vi "Save Documentation to VIs.vi"(8 "error in":errorcluster, 10 "VI Information Array":T1[](array[typedef]), 11 "Engine in":refnum<class "Engine.lvclass">) -> (0 "error out":errorcluster, 3 "Engine out":refnum<class "Engine.lvclass">)   [LabVIEW 2017, in "Engine.lvclass"]
uses:
  Engine.lvclass
  VI Information.ctl
  Engine.lvclass/Engine.ctl
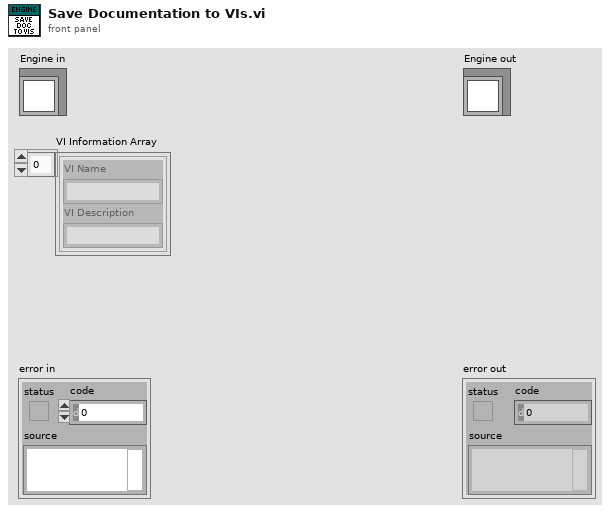
[diagram p1: front panel]
types:
  T1 = typedef "Engine.lvclass/VI Information.ctl" = cluster{"VI Name":string, "VI Description":string}
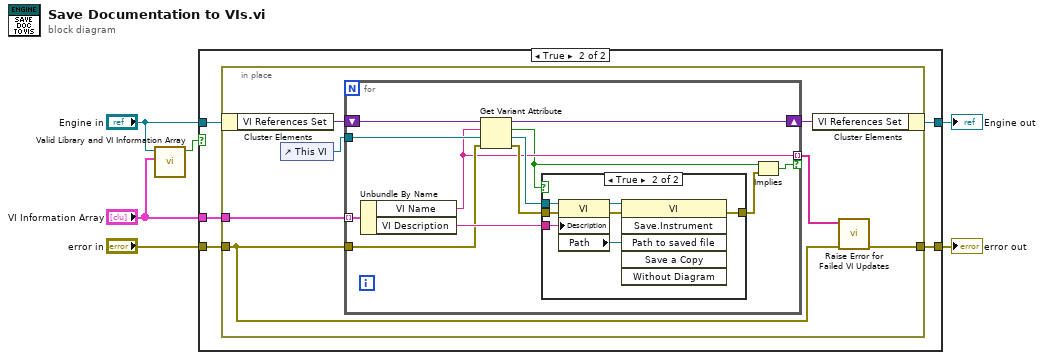
[diagram p0: block diagram]
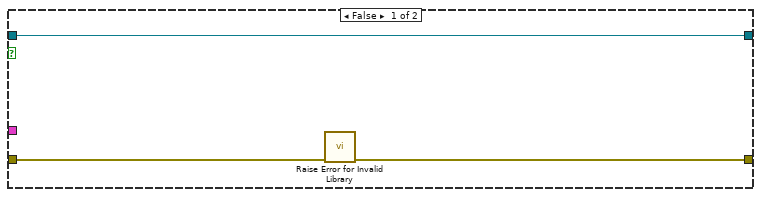
[diagram p2: hidden frame]
diagram:
  n1 = call "Valid Library and VI Information Array.vi"("VI Information Array"="VI Information Array", "Engine in"="Engine in") -> ("Valid"=w6:bool)  [unwired: 9 in]
  n2 = case shown="True" w6 {
    tunnel: [w7 w10] -> w5
    tunnel: "error in" -> [w8 w11]
    tunnel: [w9 w13] -> w3
    tunnel: "Engine in" -> [w9 w14]
    tunnel: "VI Information Array" -> [_ w12]
    frame False {
      n3 = call "Raise Error for Invalid Library.vi"("error in"=w8) -> ("error out"=w7:errorcluster)  [unwired: 10 in]
    }
    frame True {
      n4 = in-place {
        in-place-border: w12 -> [w19]
        in-place-border: w11 -> [w17]
        in-place-border: [w16] -> w10
        n5 = in-place-cluster #1(w14) -> ("VI References Set"=w20:variant)
        n6 = control-ref of="This VI"() -> (w18:refnum<vi>)
        n7 = for {
          shift-right: [w32] -> w21
          shift-left: w20 -> [w33]
          tunnel: w19 -> [w31] mode=indexing
          tunnel: w18 -> [w30]
          tunnel: w17 -> [w26]
          tunnel: [w25] -> w15 mode=indexing if=w22
          n8 = Unbundle By Name(w31) -> ("VI Name"=w25:string, "VI Description"=w28:string)
          n9 = Get Variant Attribute(Variant=w33, name=w25, default value (empty Variant)=w30, error in=w26) -> (duplicate Variant=w32:variant, found=w24:bool, value=w29:refnum<vi>, error out=w27:errorcluster)
          n10 = case shown="True" w24 {
            tunnel: w29 -> [_ w41]
            tunnel: w28 -> [_ w40]
            tunnel: w27 -> [w34 w39]
            tunnel: [w34 w35] -> w23
            frame False {
            }
            frame True {
              n11 = property class="VI"(reference=w41, error in=w39, "Description"=w40) -> (reference out=w38:refnum<vi>, error out=w37:errorcluster, "Path"=w36:path)
              n12 = invoke class="VI" method="Save.Instrument"(reference=w38, error in=w37, "Path to saved file"=w36) -> (error out=w35:errorcluster)  [unwired: 3 in, 5 out]
            }
          }
          n13 = Implies(1:w23, 2:w24) -> (0:w22:bool)
        }
        n14 = in-place-cluster #1("VI References Set"=w21) -> (w13:refnum<class "Engine.lvclass">)
        n15 = call "Raise Error for Failed VI Updates.vi"("error in"=w17, "Failed VIs"=w15) -> ("error out"=w16:errorcluster)  [unwired: 9 in]
      }
    }
  }
  "error out" <- w5
  "Engine out" <- w3
